vi "HJ212-2017.vi"(8 "error in (no error)":errorcluster caption="错误输入（无错误）", 10 "PWD？":bool, 11 "数据段":T1) -> (0 "error out":errorcluster caption="错误输出", 2 "通讯包字符串":string, 3 "通讯包":T2={"包头（2）"="##", "数据段长度（4）"="", "数据段"="", "CRC校验"="", "包尾"=""})   [LabVIEW 2016, in "数据传输系统-02.lvlib"]
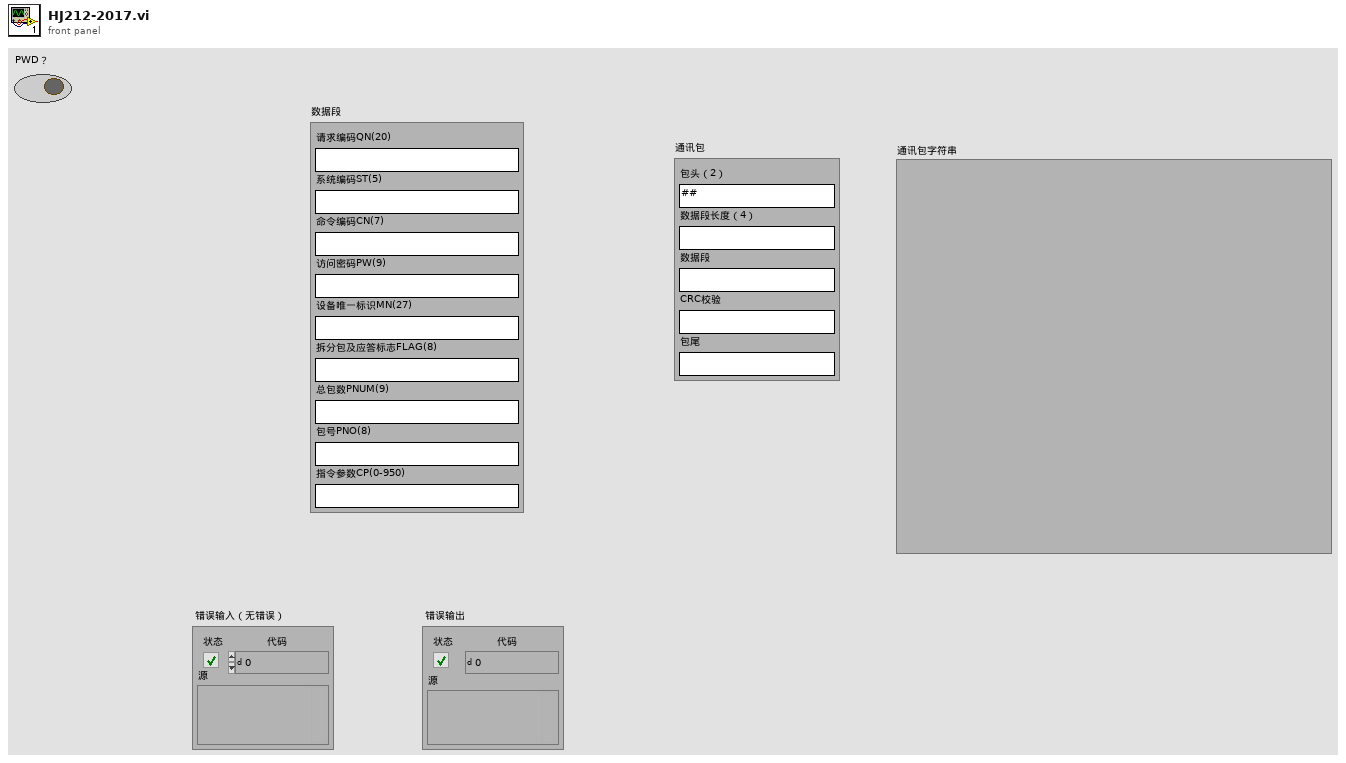
[diagram p1: front panel]
types:
  T1 = cluster{"请求编码QN(20)":string, "系统编码ST(5)":string, "命令编码CN(7)":string, "访问密码PW(9)":string, "设备唯一标识MN(27)":string, "拆分包及应答标志FLAG(8)":string, "总包数PNUM(9)":string, "包号PNO(8)":string, "指令参数CP(0-950)":string}
  T2 = cluster{"包头（2）":string, "数据段长度（4）":string, "数据段":string, "CRC校验":string, "包尾":string}
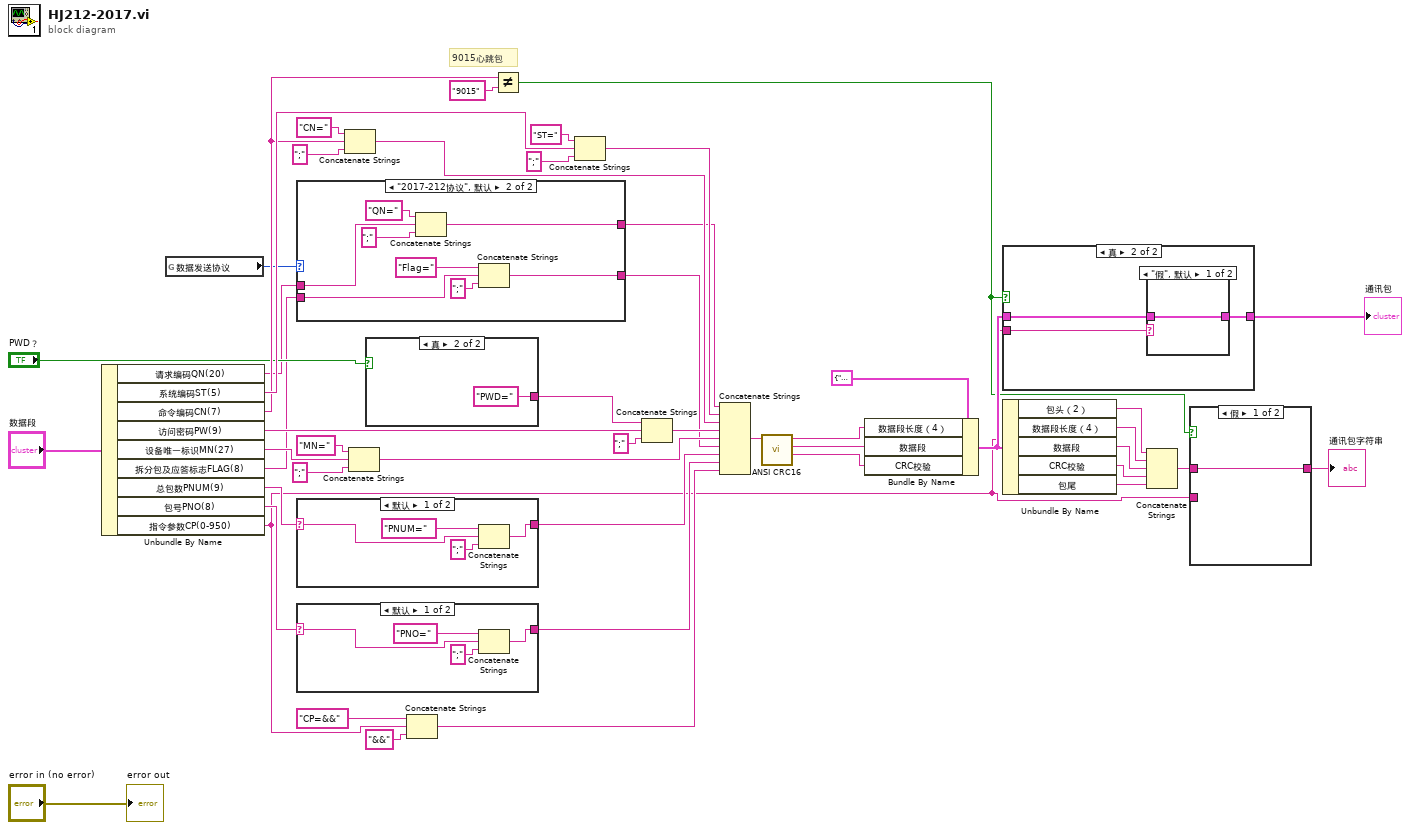
[diagram p0: block diagram]
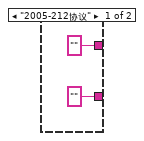
[diagram p2: hidden frame]
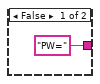
[diagram p3: hidden frame]
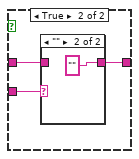
[diagram p4: hidden frame]
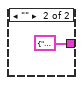
[diagram p7: hidden frame]
diagram:
  # "9015心跳包"
  n1 = Unbundle By Name("数据段") -> ("请求编码QN(20)"=w5:string, "系统编码ST(5)"=w47:string, "命令编码CN(7)"=w10:string, "访问密码PW(9)"=w43:string, "设备唯一标识MN(27)"=w41:string, "拆分包及应答标志FLAG(8)"=w3:string, "总包数PNUM(9)"=w33:string, "包号PNO(8)"=w31:string, "指令参数CP(0-950)"=w11:string)
  n2 = global read "断电保存全局.vi" "数据发送协议"() -> (w1:enum16{"2005-212协议", "2017-212协议"})
  n3 = case shown="\"2017-212协议\", 默认" w1 {
    tunnel: w5 -> [_ w54]
    tunnel: ["" w53] -> w4
    tunnel: w3 -> [_ w52]
    tunnel: ["" w51] -> w2
    frame "2005-212协议" {
    }
    frame "2017-212协议", Default {
      n4 = Concatenate Strings("QN=" ("字符串"), w54, ";" ("字符串")) -> (w53:string)
      n5 = Concatenate Strings("Flag=" ("字符串"), w52, ";" ("字符串")) -> (w51:string)
    }
  }
  n6 = case shown="默认" w33 {
    selector: w33 -> [w61 w63]
    tunnel: [w59 w63] -> w32
    frame Default {
      n7 = Concatenate Strings("PNUM=" ("字符串"), w61, ";" ("字符串")) -> (w59:string)
    }
    frame "" {
    }
  }
  n8 = case shown="默认" w31 {
    selector: w31 -> [w66 w68]
    tunnel: [w64 w68] -> w30
    frame Default {
      n9 = Concatenate Strings("PNO=" ("字符串"), w66, ";" ("字符串")) -> (w64:string)
    }
    frame "" {
    }
  }
  n10 = Concatenate Strings("CN=" ("字符串"), w10, ";" ("字符串")) -> (w37:string)
  n11 = Concatenate Strings("MN=" ("字符串"), w41, ";" ("字符串")) -> (w35:string)
  n12 = case shown="真" "PWD？" {
    tunnel: ["PW=" ("字符串") "PWD=" ("字符串")] -> w6
    frame False {
    }
    frame True {
    }
  }
  n13 = Concatenate Strings("CP=&&" ("字符串"), w11, "&&" ("字符串")) -> (w27:string)
  n14 = Not Equal?(x=w10, y="9015") -> (x != y?=w8:bool)
  n15 = Concatenate Strings("ST=" ("字符串"), w47, ";" ("字符串")) -> (w38:string)
  n16 = Concatenate Strings(w6, w43, ";" ("字符串")) -> (w36:string)
  n17 = Concatenate Strings(w4, w38, w37, w36, w35, w2, w32, w30, w27) -> (w26:string)
  n18 = call "ANSI CRC16.vi"("puchMsg"=w26) -> ("CRC校验"=w16:string, "数据段"=w17:string, "数据段长度"=w18:string)  [unwired: 8 in]
  n19 = Bundle By Name(cluster=T2 {"包头（2）"="##", "数据段长度（4）"="", "数据段"="", "CRC校验"="", "包尾"="\r\n"} ("通讯包"), "数据段长度（4）"=w18, "数据段"=w17, "CRC校验"=w16) -> (w13:T2)
  n20 = case shown="真" w8 {
    tunnel: w13 -> [w71 w74]
    tunnel: [w71 w73] -> w12
    tunnel: w11 -> [_ w72]
    frame False {
    }
    frame True {
      n21 = case shown="\"假\", 默认" w72 {
        tunnel: [w75 T2 {"包头（2）"="", "数据段长度（4）"="", "数据段"="", "CRC校验"="", "包尾"=""} ("通讯包")] -> w73
        tunnel: w74 -> [w75 _]
        frame "假", Default {
        }
        frame "" {
        }
      }
    }
  }
  "通讯包" <- w12
  n22 = Unbundle By Name(w13) -> ("包头（2）"=w23:string, "数据段长度（4）"=w22:string, "数据段"=w21:string, "CRC校验"=w20:string, "包尾"=w19:string)
  n23 = Concatenate Strings(w23, w22, w21, w20, w19) -> (w15:string)
  n24 = case shown="假" w8 {
    tunnel: w15 -> [w77 w80]
    tunnel: [w77 w79] -> w14
    tunnel: w11 -> [_ w78]
    frame False {
    }
    frame True {
      n25 = case shown="\"\"" w78 {
        tunnel: [w81 ""] -> w79
        tunnel: w80 -> [w81 _]
        frame "假", Default {
        }
        frame "" {
        }
      }
    }
  }
  "通讯包字符串" <- w14
  "error out" <- "error in (no error)"
